vi "Calculate Calibration Coefficients.vi"(7 "Channel (1)":i32=1, 8 "error in (no error)":errorcluster, 11 "VISA resource name":refnum<visa-resource-name>) -> (0 "error out":errorcluster, 3 "VISA resource name out":refnum<visa-resource-name>)   [LabVIEW 2012, in "Tektronix TTR500 Series.lvlib"]
doc: "From the measured calibration data, calculates the calibration coefficients depending on the selected calibration type.\nCalculating the calibration coefficients clears all calibration data whether or not used for the calculation and also clears the calibration type selections.\n\nNotes:\nIf you execute this function before all necessary calibration data for calculating the calibration coefficients is measured, an error occurs and the function is ignored."
uses:
  <instrlib>/Tektronix TTR500 Series/Tektronix TTR500 Series.lvlib
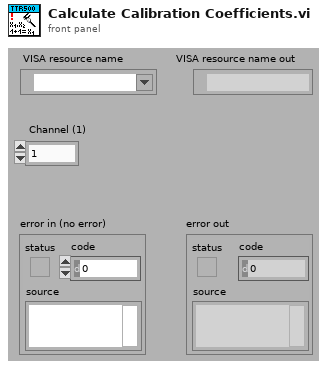
[diagram p1: front panel]
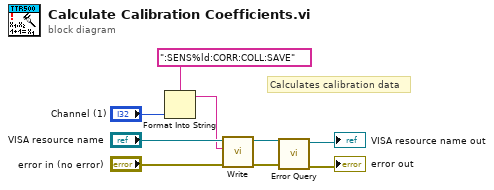
[diagram p0: block diagram]
diagram:
  # "Calculates calibration data"
  n1 = Format Into String(format string=":SENS%ld:CORR:COLL:SAVE", "Channel (1)") -> (resulting string=w6:string)  [unwired: 2 in, 1 out]
  n2 = call <instrlib>:"Write.vi"("error in (no error)"="error in (no error)", "String ()"=w6, "VISA resource name"="VISA resource name") -> ("error out"=w3:errorcluster, "VISA resource name out"=w4:refnum<visa-resource-name>)  [unwired: 6 in, 1 out]
  n3 = call <instrlib>:"Error Query.vi"("error in (no error)"=w3, "VISA resource name"=w4) -> ("error out"=→"error out":errorcluster, "VISA resource name out"=→"VISA resource name out":refnum<visa-resource-name>)  [unwired: 6 in, 2 out]
